vi "Check PXIe-433x Presence.vi"(8 "error in (no error)":errorcluster) -> (0 "error out":errorcluster, 2 "PXIe-433x Present?":bool, 3 "PXIe-433x Resources":tag[](array[tag]))   [LabVIEW 2011, in "PXIe-433x Custom Device.lvlib"]
uses:
  PXIe-433x Custom Device.lvlib
  Program Files (x86)/National Instruments/LabVIEW 2011/resource/objmgr/daqmx.rc
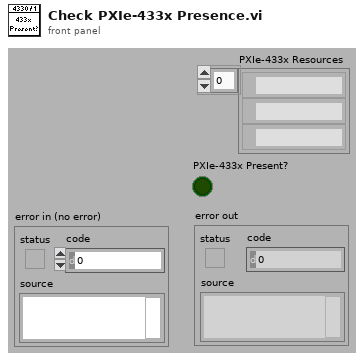
[diagram p1: front panel]
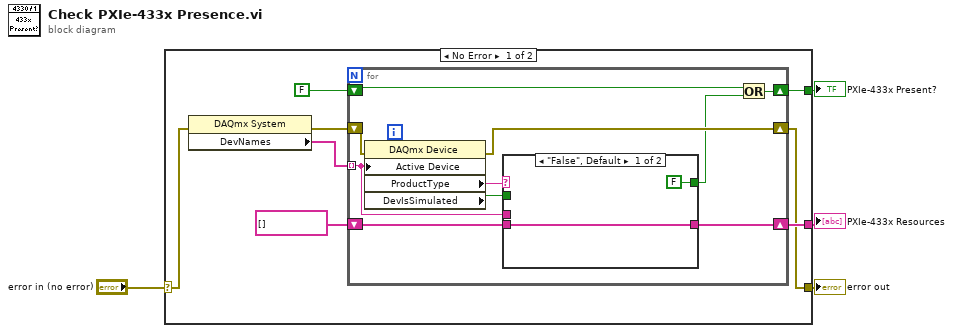
[diagram p0: block diagram]
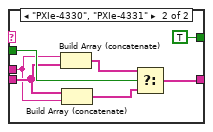
[diagram p2: hidden frame]
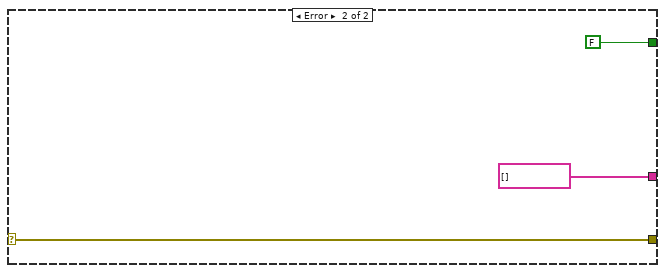
[diagram p3: hidden frame]
diagram:
  n1 = case shown="No Error" "error in (no error)" {
    selector: "error in (no error)" -> [w8 w34]
    tunnel: [w9 tag[] []] -> w4
    tunnel: [w7 w34] -> w2
    tunnel: [w5 FALSE] -> w1
    frame No Error {
      n2 = property class="DAQmx System"(error in=w8) -> (error out=w10:errorcluster, "DevNames"=w12:tag[])  [unwired: 1 in, 1 out]
      n3 = for {
        tunnel: w12 -> [w13] mode=indexing
        shift-right: [w18] -> w9
        shift-left: tag[] [] -> [w19]
        shift-right: [w21] -> w7
        shift-left: w10 -> [w22]
        shift-right: [w17] -> w5
        shift-left: FALSE -> [w16]
        n4 = property class="DAQmx Device"(error in=w22, "Active Device"=w13) -> (error out=w21:errorcluster, "ProductType"=w20:string, "DevIsSimulated"=w15:bool)  [unwired: 1 in, 1 out]
        n5 = case shown="\"False\", Default" w20 {
          tunnel: [FALSE TRUE] -> w14
          tunnel: w19 -> [w24 w27]
          tunnel: [w24 w29] -> w18
          tunnel: w15 -> [_ w30]
          tunnel: w13 -> [_ w26]
          frame "False", Default {
          }
          frame "PXIe-4330", "PXIe-4331" {
            n6 = Build Array (concatenate)(w26, w27) -> (w28:tag[])
            n7 = Build Array (concatenate)(w27, w26) -> (w25:tag[])
            n8 = Select(t=w28, s=w30, f=w25) -> (s? t:f=w29:tag[])
          }
        }
        n9 = Or(x=w16, y=w14) -> (x .or. y?=w17:bool)
      }
    }
    frame Error {
    }
  }
  "error out" <- w2
  "PXIe-433x Resources" <- w4
  "PXIe-433x Present?" <- w1
